vi "UI_Gear_Unit_Test.vi"() -> ()   [LabVIEW 2014]
panel:
  out "轴承温度异常":bool
  out "齿轮箱轴承温度8":dbl
  out "齿轮箱轴承温度7":dbl
  out "齿轮箱轴承温度6":dbl
  out "齿轮箱轴承温度5":dbl
  out "齿轮箱轴承温度4":dbl
  out "齿轮箱轴承温度3":dbl
  out "齿轮箱轴承温度2":dbl
  out "齿轮箱轴承温度1":dbl
  out "油站系统综合状态异常":bool
  out "油箱系统综合状态":bool caption="油站系统综合状态"
  out "供油流量状态":bool
  out "散热器风机状态":bool
  out "回油泵状态":bool
  out "2号油泵状态":bool
  out "1号油泵状态":bool
  out "齿轮箱油站调试状态":bool
  in  "退出":bool
  in  "开始调试":bool
  in  "供油流量异常":bool
  in  "供油压力异常":bool
  in  "齿轮子系统2号油泵故障":bool caption="2号油泵故障"
  in  "齿轮子系统1号油泵故障":bool caption="1号油泵故障"
  in  "回油泵故障":bool
  in  "齿轮子系统循环回路过滤器压差过高":bool caption="散热器风机故障"
  in  "齿轮子系统供油过滤器压差过高":bool caption="供油过滤器压差过高"
  in  "供油油温异常":bool
  in  "齿轮子系统油箱液位过低":bool caption="油箱液位过低"
  in  "齿轮子系统油箱液位过高":bool caption="油箱液位过高"
  in  "齿轮子系统加热装置异常":bool caption="油箱加热器异常"
  out "供油油温":dbl(graph)
  out "过滤器压差":bool
  out "供油压力":dbl(graph)
  out "油箱润滑油液位":bool
  out "油箱温度":dbl(graph)
  # "齿轮箱油站独立调试"
  # "监测参数"
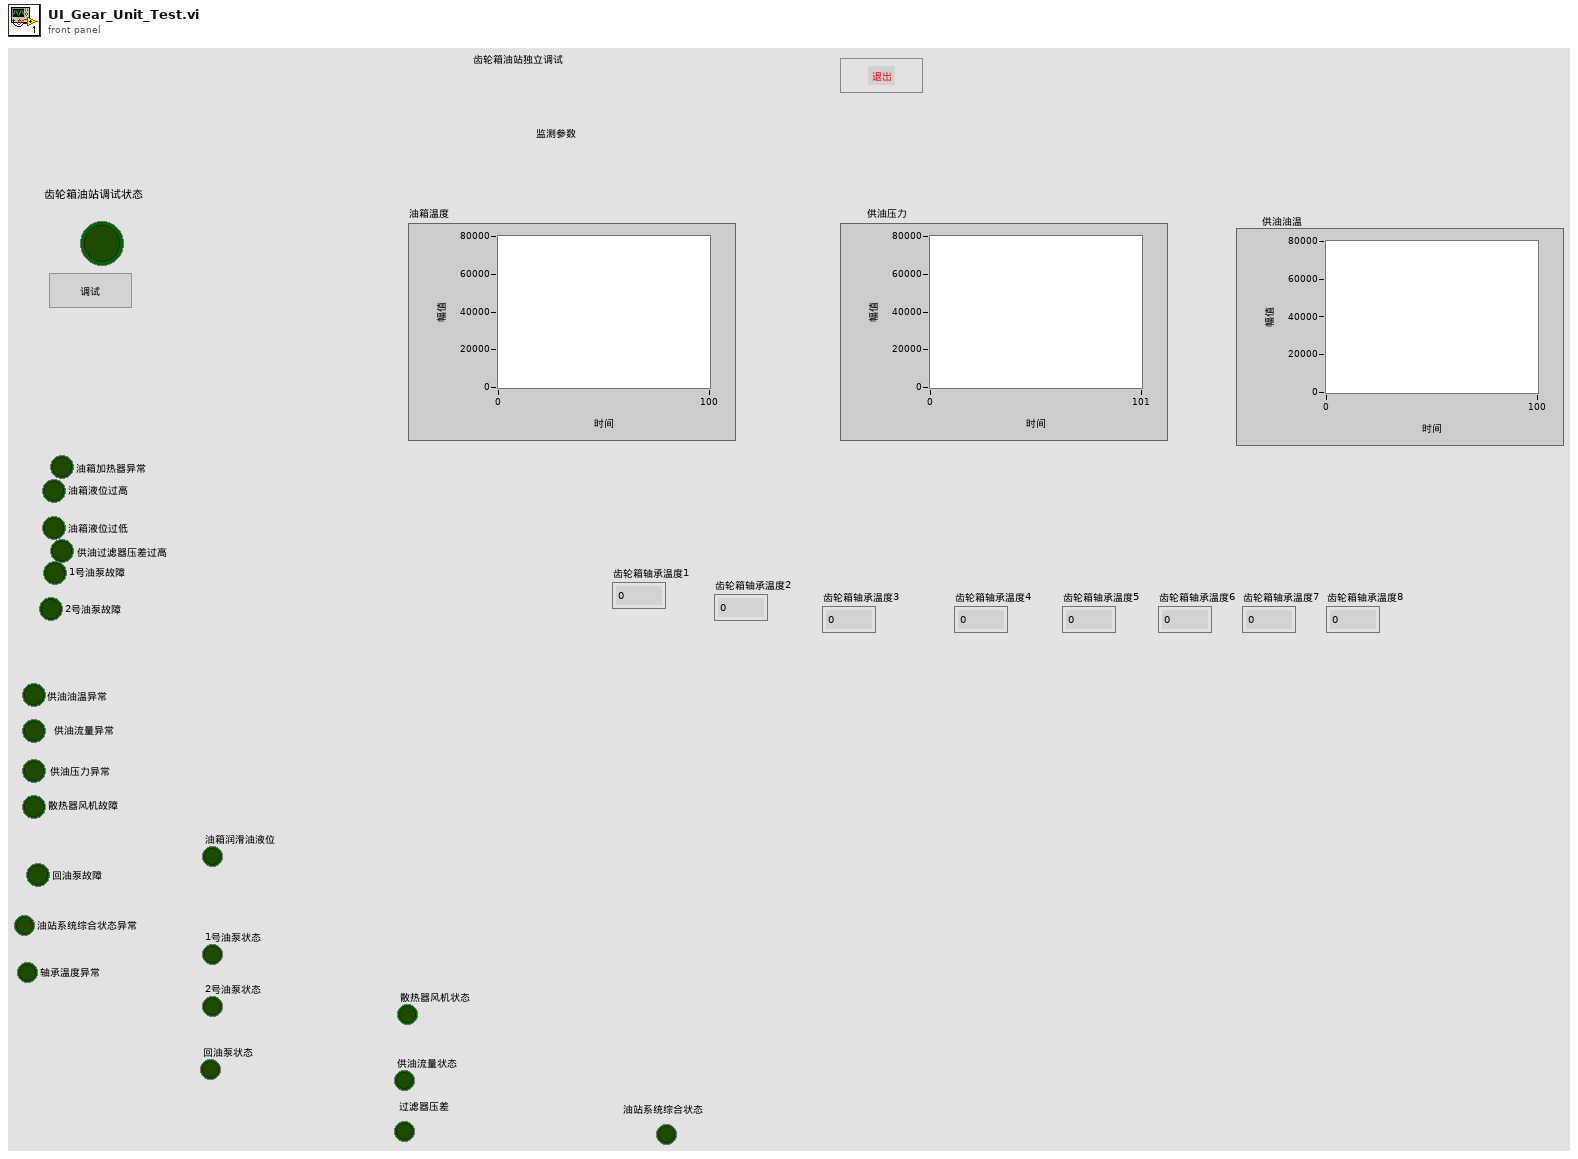
[diagram p1: front panel]
types:
  T1 = cluster{"油箱温度":u16, "供油油温":u16, "供油压力":u16, "油箱润滑油液位":bool, "1号油泵状态":bool, "2号油泵状态":bool, "回油泵状态":bool, "散热器风机状态":bool, "供油流量状态":bool, "过滤器压差":bool, "油箱系统综合状态":bool, "齿轮箱轴承温度1":u16, "齿轮箱轴承温度2":u16, "齿轮箱轴承温度3":u16, "齿轮箱轴承温度4":u16, "齿轮箱轴承温度5":u16, "齿轮箱轴承温度6":u16, "齿轮箱轴承温度7":u16, "齿轮箱轴承温度8":u16, "齿轮子系统状态字":cluster{"油箱加热器异常故障报警":bool, "油箱液位过高报警":bool, "油箱液位过低报警":bool, "供油过滤器压差过高报警":bool, "1号油泵故障报警":bool, "2号油泵故障报警":bool, "回油泵故障报警":bool, "散热器风机故障报警":bool, "供油压力异常报警":bool, "供油流量异常报警":bool, "供油油温异常报警":bool, "油站系统综合状态异常报警":bool, "轴承温度异常报警":bool}}
  T2 = cluster{"油箱加热器异常故障报警":bool, "油箱液位过高报警":bool, "油箱液位过低报警":bool, "供油过滤器压差过高报警":bool, "1号油泵故障报警":bool, "2号油泵故障报警":bool, "回油泵故障报警":bool, "散热器风机故障报警":bool, "供油压力异常报警":bool, "供油流量异常报警":bool, "供油油温异常报警":bool, "油站系统综合状态异常报警":bool, "轴承温度异常报警":bool}
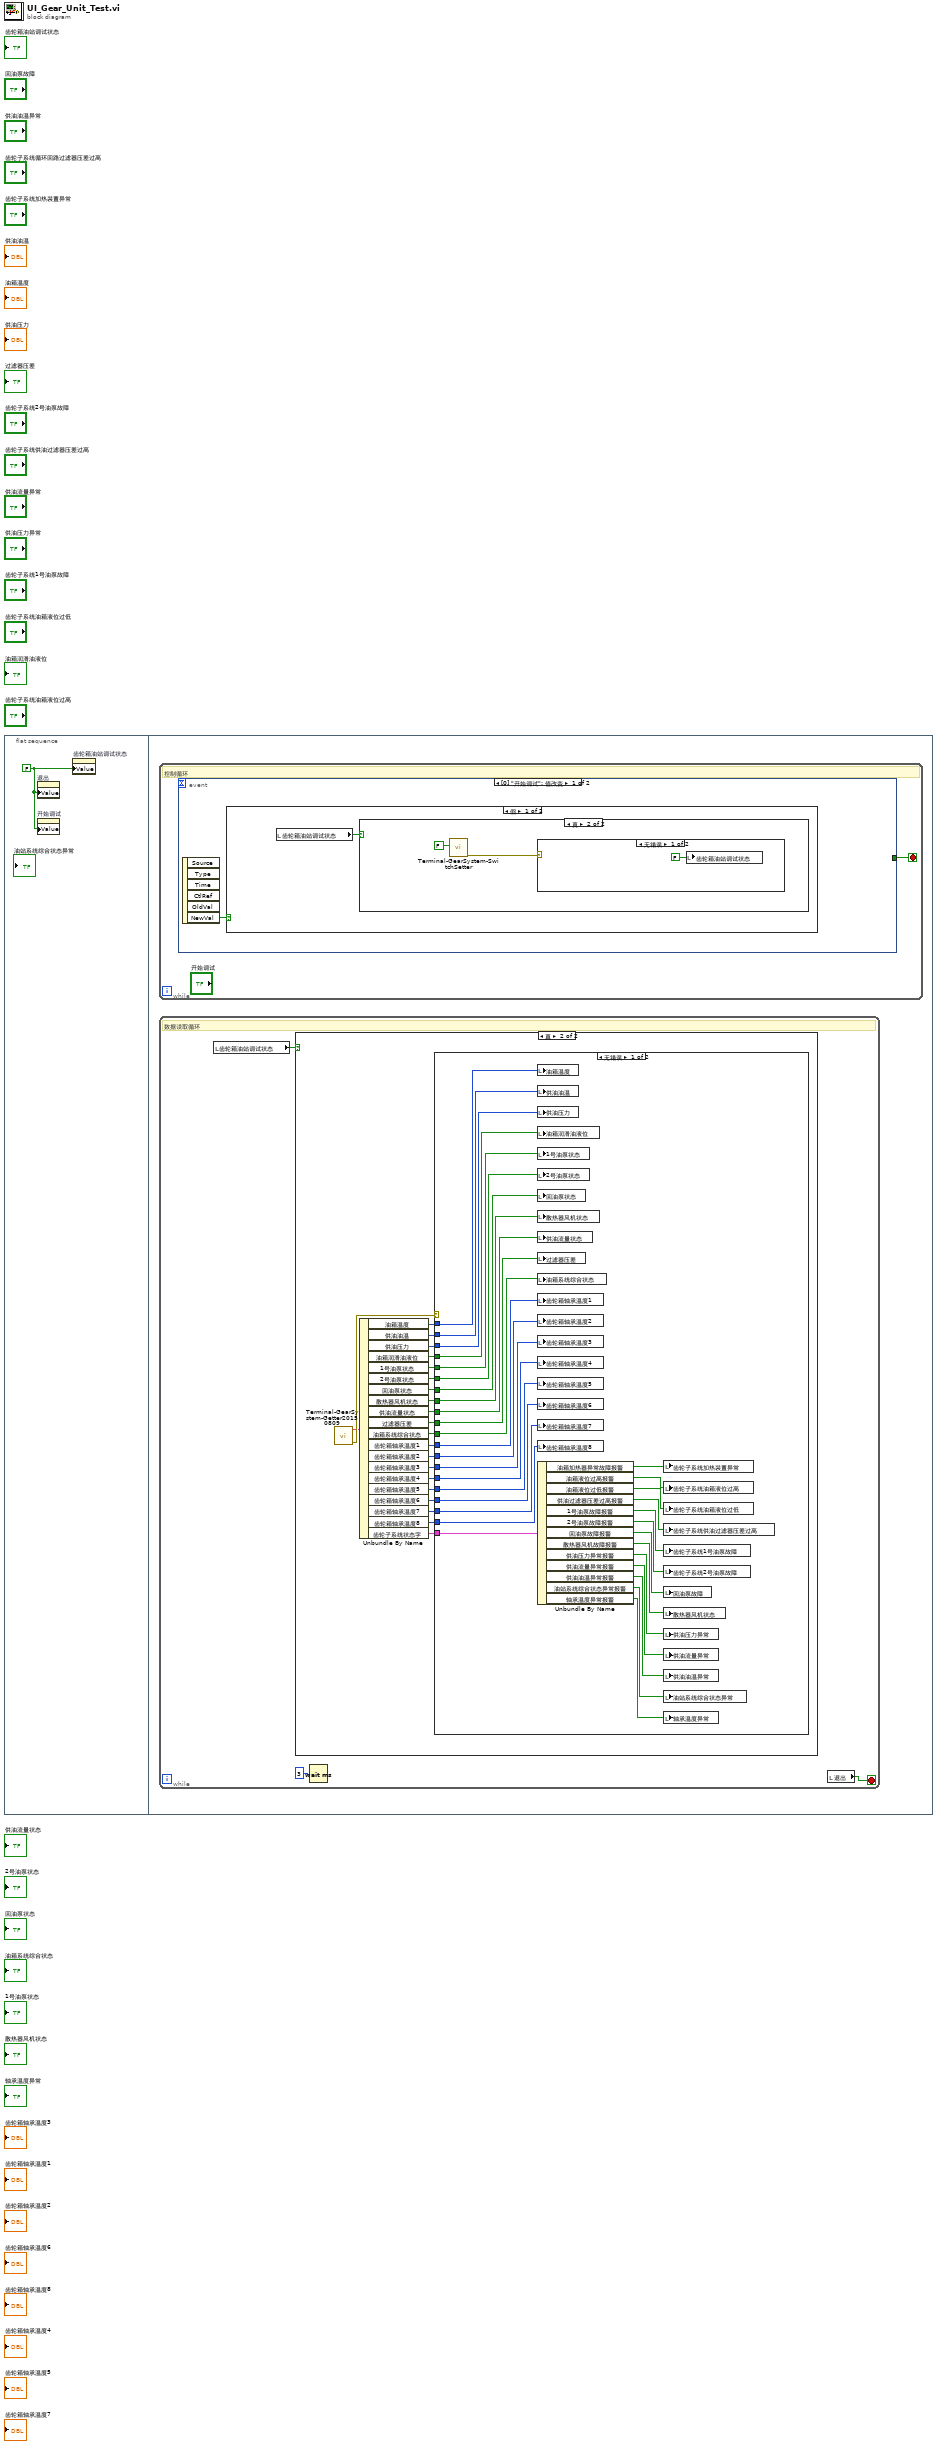
[diagram p0: block diagram]
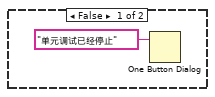
[diagram p4: hidden frame]
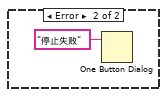
[diagram p5: hidden frame]
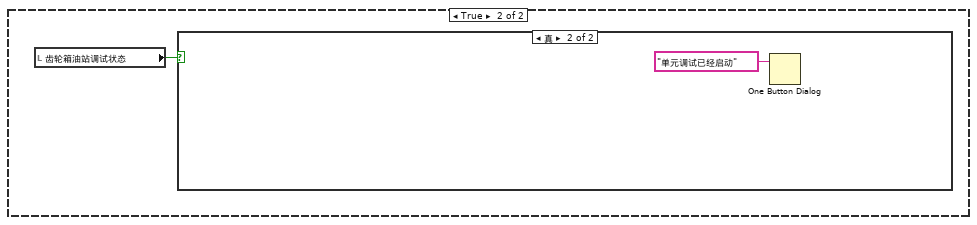
[diagram p6: hidden frame]
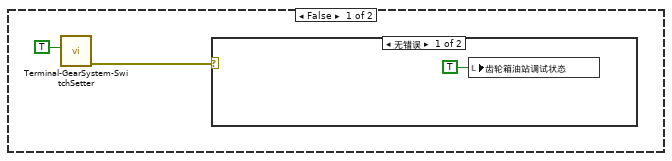
[diagram p7: hidden frame]
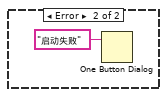
[diagram p8: hidden frame]
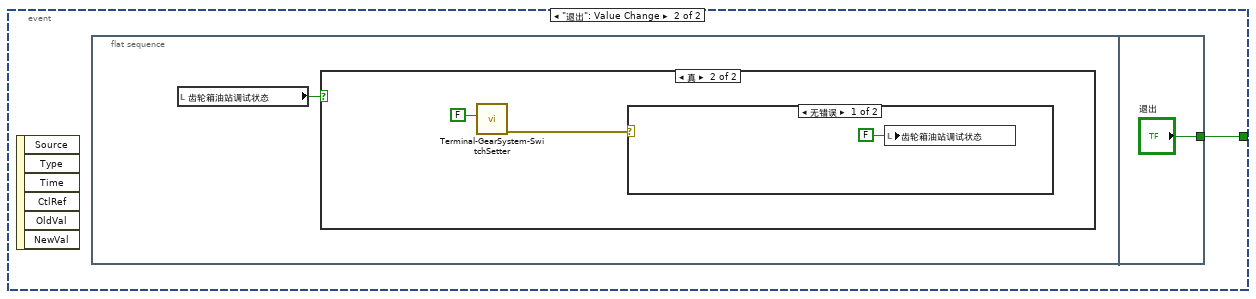
[diagram p9: hidden frame]
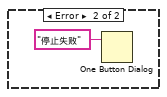
[diagram p11: hidden frame]
diagram:
  n1 = flat-sequence {
    frame #0 {
      w1 = FALSE ("齿轮箱油站调试状态")
      n2 = property on="退出" class="Bool (严格)"("Value"=w1) -> ()  [unwired: 2 in, 2 out]
      n3 = property on="开始调试" class="Bool (严格)"("Value"=w1) -> ()  [unwired: 2 in, 2 out]
      n4 = property on="齿轮箱油站调试状态" class="Bool (严格)"("Value"=w1) -> ()  [unwired: 2 in, 2 out]
    }
    frame #1 {
      n5 = while {
        stop <- w60 stop-if-true
        # "控制循环"
        n6 = event shown="[0] \"开始调试\": 值改变" {
          selector: _ -> [_ _]
          dyn-events: _ -> [_ _]
          timeout: _ -> [_ _]
          tunnel: [_ w74] -> w60
          event "开始调试": Value Change {
            n7 = event-data() -> ("NewVal"=w61:bool)  [unwired: 1 in, 5 out]
            n8 = case shown="假" w61 {
              frame False {
                n9 = local read "齿轮箱油站调试状态"() -> (w62:bool)
                n10 = case shown="真" w62 {
                  frame False {
                    n11 = One Button Dialog(message="单元调试已经停止" ("消息")) -> ()  [unwired: 1 in, 1 out]
                  }
                  frame True {
                    n12 = call "Terminal-GearSystem-SwitchSetter.vi"("启停"=FALSE) -> ("error out"=w64:errorcluster)  [unwired: 10 in]
                    n13 = case shown="无错误" w64 {
                      frame No Error {
                        n14 = local write "齿轮箱油站调试状态"(FALSE) -> ()
                      }
                      frame Error {
                        n15 = One Button Dialog(message="停止失败" ("消息")) -> ()  [unwired: 1 in, 1 out]
                      }
                    }
                  }
                }
              }
              frame True {
                n16 = local read "齿轮箱油站调试状态"() -> (w68:bool)
                n17 = case shown="真" w68 {
                  frame False {
                    n18 = call "Terminal-GearSystem-SwitchSetter.vi"("启停"=TRUE) -> ("error out"=w69:errorcluster)  [unwired: 10 in]
                    n19 = case shown="无错误" w69 {
                      frame No Error {
                        n20 = local write "齿轮箱油站调试状态"(TRUE) -> ()
                      }
                      frame Error {
                        n21 = One Button Dialog(message="启动失败" ("消息")) -> ()  [unwired: 1 in, 1 out]
                      }
                    }
                  }
                  frame True {
                    n22 = One Button Dialog(message="单元调试已经启动" ("消息")) -> ()  [unwired: 1 in, 1 out]
                  }
                }
              }
            }
          }
          event "退出": Value Change {
            n23 = event-data() -> ()  [unwired: 1 in, 6 out]
            n24 = flat-sequence {
              tunnel: ["退出"] -> w74
              frame #0 {
                n25 = local read "齿轮箱油站调试状态"() -> (w75:bool)
                n26 = case shown="真" w75 {
                  frame False {
                  }
                  frame True {
                    n27 = call "Terminal-GearSystem-SwitchSetter.vi"("启停"=FALSE) -> ("error out"=w77:errorcluster)  [unwired: 10 in]
                    n28 = case shown="无错误" w77 {
                      frame No Error {
                        n29 = local write "齿轮箱油站调试状态"(FALSE) -> ()
                      }
                      frame Error {
                        n30 = One Button Dialog(message="停止失败" ("消息")) -> ()  [unwired: 1 in, 1 out]
                      }
                    }
                  }
                }
              }
              frame #1 {
              }
            }
          }
        }
      }
      n31 = while {
        stop <- w3 stop-if-true
        # "数据读取循环"
        n32 = local read "齿轮箱油站调试状态"() -> (w4:bool)
        n33 = case shown="真" w4 {
          frame False {
          }
          frame True {
            n34 = call "Terminal-GearSystem-Getter20150809.vi"() -> ("error out"=w26:errorcluster, "设备信息"=w25:T1)  [unwired: 9 in, 1 out]
            n35 = Unbundle By Name(w25) -> ("油箱温度"=w23:u16, "供油油温"=w22:u16, "供油压力"=w21:u16, "油箱润滑油液位"=w20:bool, "1号油泵状态"=w19:bool, "2号油泵状态"=w18:bool, "回油泵状态"=w17:bool, "散热器风机状态"=w16:bool, "供油流量状态"=w15:bool, "过滤器压差"=w14:bool, "油箱系统综合状态"=w13:bool, "齿轮箱轴承温度1"=w12:u16, "齿轮箱轴承温度2"=w11:u16, "齿轮箱轴承温度3"=w10:u16, "齿轮箱轴承温度4"=w9:u16, "齿轮箱轴承温度5"=w8:u16, "齿轮箱轴承温度6"=w7:u16, "齿轮箱轴承温度7"=w6:u16, "齿轮箱轴承温度8"=w5:u16, "齿轮子系统状态字"=w24:T2)
            n36 = case shown="无错误" w26 {
              tunnel: w24 -> [w59 _]
              tunnel: w23 -> [w45 _]
              tunnel: w22 -> [w44 _]
              tunnel: w21 -> [w43 _]
              tunnel: w20 -> [w42 _]
              tunnel: w19 -> [w41 _]
              tunnel: w18 -> [w40 _]
              tunnel: w17 -> [w39 _]
              tunnel: w16 -> [w38 _]
              tunnel: w15 -> [w37 _]
              tunnel: w14 -> [w36 _]
              tunnel: w13 -> [w35 _]
              tunnel: w12 -> [w34 _]
              tunnel: w11 -> [w33 _]
              tunnel: w10 -> [w32 _]
              tunnel: w9 -> [w31 _]
              tunnel: w8 -> [w30 _]
              tunnel: w7 -> [w29 _]
              tunnel: w6 -> [w28 _]
              tunnel: w5 -> [w27 _]
              frame No Error {
                n37 = local write "油箱温度"(w45) -> ()
                n38 = local write "供油油温"(w44) -> ()
                n39 = local write "供油压力"(w43) -> ()
                n40 = local write "油箱润滑油液位"(w42) -> ()
                n41 = local write "1号油泵状态"(w41) -> ()
                n42 = local write "2号油泵状态"(w40) -> ()
                n43 = local write "回油泵状态"(w39) -> ()
                n44 = local write "散热器风机状态"(w38) -> ()
                n45 = local write "供油流量状态"(w37) -> ()
                n46 = local write "过滤器压差"(w36) -> ()
                n47 = local write "油箱系统综合状态"(w35) -> ()
                n48 = local write "齿轮箱轴承温度1"(w34) -> ()
                n49 = local write "齿轮箱轴承温度2"(w33) -> ()
                n50 = local write "齿轮箱轴承温度3"(w32) -> ()
                n51 = local write "齿轮箱轴承温度4"(w31) -> ()
                n52 = local write "齿轮箱轴承温度5"(w30) -> ()
                n53 = local write "齿轮箱轴承温度6"(w29) -> ()
                n54 = local write "齿轮箱轴承温度7"(w28) -> ()
                n55 = local write "齿轮箱轴承温度8"(w27) -> ()
                n56 = Unbundle By Name(w59) -> ("油箱加热器异常故障报警"=w58:bool, "油箱液位过高报警"=w57:bool, "油箱液位过低报警"=w56:bool, "供油过滤器压差过高报警"=w55:bool, "1号油泵故障报警"=w54:bool, "2号油泵故障报警"=w53:bool, "回油泵故障报警"=w52:bool, "散热器风机故障报警"=w51:bool, "供油压力异常报警"=w50:bool, "供油流量异常报警"=w49:bool, "供油油温异常报警"=w48:bool, "油站系统综合状态异常报警"=w47:bool, "轴承温度异常报警"=w46:bool)
                n57 = local write "齿轮子系统加热装置异常"(w58) -> ()
                n58 = local write "齿轮子系统油箱液位过高"(w57) -> ()
                n59 = local write "齿轮子系统油箱液位过低"(w56) -> ()
                n60 = local write "齿轮子系统供油过滤器压差过高"(w55) -> ()
                n61 = local write "齿轮子系统1号油泵故障"(w54) -> ()
                n62 = local write "齿轮子系统2号油泵故障"(w53) -> ()
                n63 = local write "回油泵故障"(w52) -> ()
                n64 = local write "散热器风机状态"(w51) -> ()
                n65 = local write "供油压力异常"(w50) -> ()
                n66 = local write "供油流量异常"(w49) -> ()
                n67 = local write "供油油温异常"(w48) -> ()
                n68 = local write "油站系统综合状态异常"(w47) -> ()
                n69 = local write "轴承温度异常"(w46) -> ()
              }
              frame Error {
              }
            }
          }
        }
        n70 = Wait (ms)(milliseconds to wait=u32 3 ("等待时间（毫秒）")) -> ()  [unwired: 1 out]
        n71 = local read "退出"() -> (w3:bool)
      }
    }
  }
